vi "锁紧试验判定.vi"(7 "Result":refnum<vi>, 10 "判定参数":T1={"手柄锁紧最大力"={"单位"="N", "下限"=1.0, "上限"=2.0}}, 11 "XY曲线":cluster{"X":dbl[], "Y":dbl[]}[](array[cluster])) -> (2 "判定项长度":i32, 3 "OK？":bool)   [LabVIEW 2020]
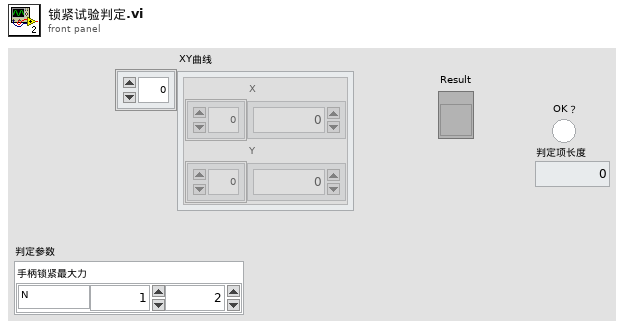
[diagram p1: front panel]
types:
  T1 = cluster{"手柄锁紧最大力":cluster{"单位":string, "下限":dbl, "上限":dbl}}
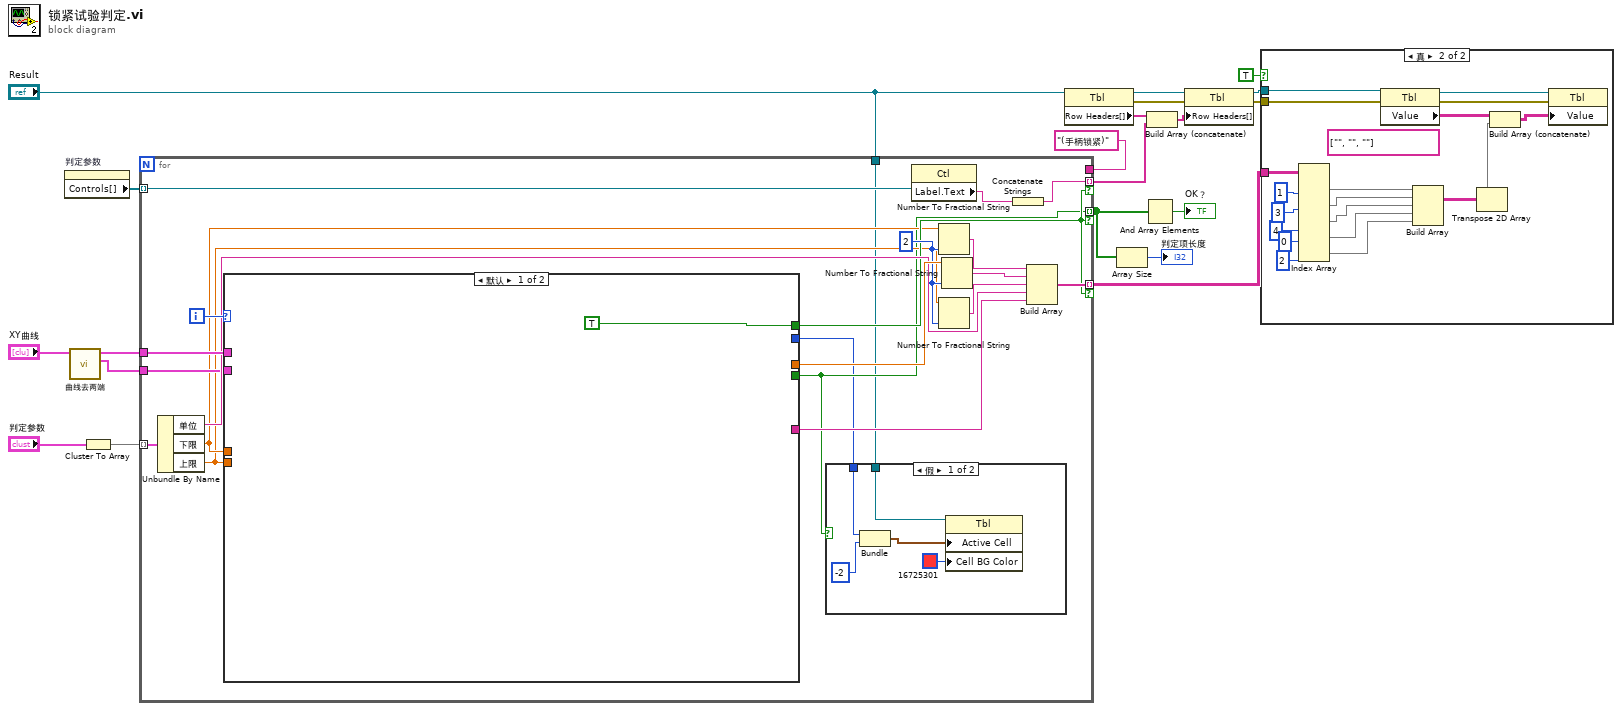
[diagram p0: block diagram]
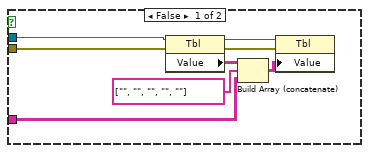
[diagram p2: hidden frame]
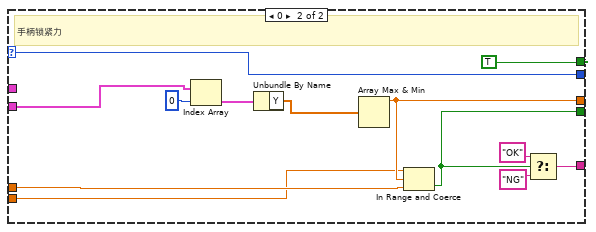
[diagram p4: hidden frame]
diagram:
  n1 = property on="判定参数" class="Clust (严格)"() -> ("Controls[]"=w11:refnum<vi>[])  [unwired: 2 in, 2 out]
  n2 = call "曲线去两端.vi"("曲线In"="XY曲线") -> ("启动曲线"=w4:cluster{"X":dbl[], "Y":dbl[]}[], "曲线Out"=w7:cluster{"X":dbl[], "Y":dbl[]}[])  [unwired: 9 in]
  n3 = Cluster To Array(cluster="判定参数") -> (array=w2:cluster{"单位":string, "下限":dbl, "上限":dbl}[])
  n4 = for {
    tunnel: w11 -> [w40] mode=indexing
    tunnel: w7 -> [w38]
    tunnel: [w23] -> w6 mode=indexing if=w29
    tunnel: [w31] -> w12 mode=indexing if=w29
    tunnel: [w25] -> w14 mode=indexing if=w29
    tunnel: w4 -> [w28]
    tunnel: "(手柄锁紧)" ("Label.Text") -> [_]
    tunnel: w2 -> [w24] mode=indexing
    tunnel: "Result" -> [w22]
    i -> [w41]
    w37 = i16 2 ("精度(6)")
    n5 = Unbundle By Name(w24) -> ("单位"=w32:string, "下限"=w27:dbl, "上限"=w26:dbl)
    n6 = case shown="默认" w41 {
      selector: w41 -> [_ w48]
      tunnel: [_ w58] -> w39
      tunnel: w38 -> [_ _]
      tunnel: [_ w55] -> w33
      tunnel: [_ w54] -> w23
      tunnel: w27 -> [_ w53]
      tunnel: w26 -> [_ w52]
      tunnel: [TRUE TRUE] -> w29
      tunnel: w28 -> [_ w49]
      tunnel: [_ w48] -> w21
      frame Default {
      }
      frame 0 {
        # "手柄锁紧力"
        n7 = Index Array(array=w49, index=0 ("索引")) -> (element=w59:cluster{"X":dbl[], "Y":dbl[]})
        n8 = Unbundle By Name(w59) -> ("Y"=w50:dbl[])
        n9 = Array Max & Min(array=w50) -> (max value=w58:dbl)  [unwired: 3 out]
        n10 = In Range and Coerce(upper limit=w52, x=w58, lower limit=w53) -> (In Range?=w54:bool)  [unwired: 1 out]
        n11 = Select(t="OK", s=w54, f="NG") -> (s? t:f=w55:string)
      }
    }
    n12 = case shown="假" w23 {
      tunnel: w22 -> [w46 _]
      tunnel: w21 -> [w44 _]
      frame False {
        n13 = Bundle(w44, "索引"=-2) -> (w43:cluster{i32, "索引":i32})  [unwired: 1 in]
        n14 = property class="Tbl"(reference=w46, "Active Cell"=w43, "Cell BG Color"=u32 16725301 ("活动单元格:单元格背景色")) -> ()  [unwired: 1 in, 2 out]
      }
      frame True {
      }
    }
    n15 = property class="Ctl"(reference=w40) -> ("Label.Text"=w30:string)  [unwired: 1 in, 2 out]
    n16 = Number To Fractional String(number=w27, precision (6)=w37) -> (F-format string=w36:string)  [unwired: 2 in]
    n17 = Number To Fractional String(number=w26, precision (6)=w37) -> (F-format string=w34:string)  [unwired: 2 in]
    n18 = Number To Fractional String(number=w39, precision (6)=w37) -> (F-format string=w35:string)  [unwired: 2 in]
    n19 = Concatenate Strings(w30) -> (w25:string)
    n20 = Build Array(w36, w35, w34, w32, w33) -> (w31:string[])
  }
  n21 = property class="Tbl"(reference="Result") -> (reference out=w16:refnum<vi>, error out=w19:errorcluster, "Row Headers[]"=w13:string[])  [unwired: 1 in]
  n22 = Array Size(array=w6) -> (size(s)=→"判定项长度":i32)
  n23 = And Array Elements(Boolean array=w6) -> (logical AND=→"OK？":bool)
  n24 = Build Array (concatenate)(w13, w14) -> (w15:string[])
  n25 = property class="Tbl"(reference=w16, error in=w19, "Row Headers[]"=w15) -> (reference out=w17:refnum<vi>, error out=w18:errorcluster)
  n26 = case shown="真" TRUE {
    tunnel: w18 -> [w66 w86]
    tunnel: w17 -> [w63 w83]
    tunnel: w12 -> [w62 w80]
    frame False {
      n27 = property class="Tbl"(reference=w63, error in=w66) -> (reference out=w64:refnum<vi>, error out=w65:errorcluster, "Value"=w67:string[][])
      n28 = Build Array (concatenate)(w67, string[] ["", "", "", "", ""], w62) -> (w68:string[][])
      n29 = property class="Tbl"(reference=w64, error in=w65, "Value"=w68) -> ()  [unwired: 2 out]
    }
    frame True {
      (unwired) string[] ["", "", ""]
      n30 = Index Array(array=w80, index (col) #1=1 ("禁用的索引 (列)"), index (col) #2=3 ("索引 (列)"), index (col) #3=4 ("索引 (列)"), index (col) #4=0 ("索引 (列)"), index (col) #5=2 ("索引 (列)")) -> (element #1=w75:string[], element #2=w74:string[], element #3=w73:string[], element #4=w72:string[], element #5=w71:string[])  [unwired: 5 in]
      n31 = property class="Tbl"(reference=w83, error in=w86) -> (reference out=w84:refnum<vi>, error out=w85:errorcluster, "Value"=w87:string[][])
      n32 = Build Array(w75, w74, w73, w72, w71) -> (w77:string[][])
      n33 = Transpose 2D Array ("二维数组转置")(2D array=w77) -> (transposed array=w69:string[][])
      n34 = Build Array (concatenate)(w87, w69) -> (w76:string[][])
      n35 = property class="Tbl"(reference=w84, error in=w85, "Value"=w76) -> ()  [unwired: 2 out]
    }
  }
